vi "add search path.vi"(8 "error in":errorcluster, 10 "search path":path, 11 "glyph manager in":T1) -> (0 "error out":errorcluster, 3 "glyph manager out":T1)   [LabVIEW 2013, in "glyph manager.lvlib"]
uses:
  glyph manager.lvlib
  glyph manager.ctl
  <vilib>/picture/picture.llb/imagedata.ctl
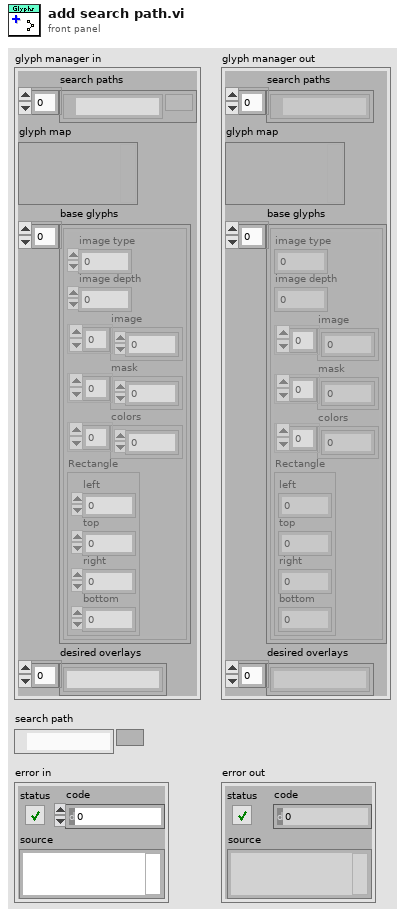
[diagram p1: front panel]
types:
  T1 = typedef "glyph manager.lvlib/glyph manager.ctl" = cluster{"search paths":path[], "glyph map":variant, "base glyphs":T2[], "desired overlays":string[]}
  T2 = typedef "imagedata.ctl" = cluster{"image type":i32, "image depth":i32, "image":u8[], "mask":u8[], "colors":u32[], "Rectangle":cluster{"left":i16, "top":i16, "right":i16, "bottom":i16}}
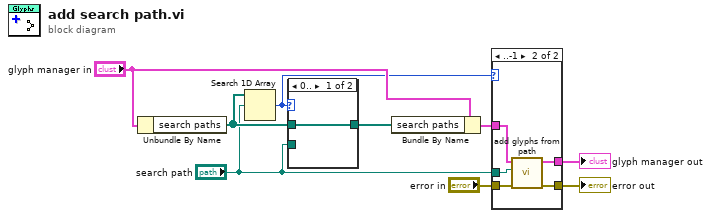
[diagram p0: block diagram]
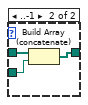
[diagram p3: hidden frame]
diagram:
  n1 = Unbundle By Name("glyph manager in") -> ("search paths"=w8:path[])
  n2 = Search 1D Array(1D array=w8, element="search path") -> (index of element=w5:i32)  [unwired: 1 in]
  n3 = case shown="0.." w5 {
    tunnel: w8 -> [w10 w13]
    tunnel: "search path" -> [_ w11]
    tunnel: [w10 w12] -> w7
    frame 0.. {
    }
    frame ..-1 {
      n4 = Build Array (concatenate)(w13, w11) -> (w12:path[])
    }
  }
  n5 = Bundle By Name(cluster="glyph manager in", "search paths"=w7) -> (w2:T1)
  n6 = case shown="..-1" w5 {
    tunnel: [w15 w20] -> w6
    tunnel: "error in" -> [w15 w19]
    tunnel: "search path" -> [_ w18]
    tunnel: w2 -> [w14 w17]
    tunnel: [w14 w16] -> w1
    frame 0.. {
    }
    frame ..-1 {
      n7 = call "add glyphs from path.vi"("error in (no error)"=w19, "Path"=w18, "glyph manager in"=w17) -> ("error out"=w20:errorcluster, "glyph manager out"=w16:T1)  [unwired: 7 in]
    }
  }
  "error out" <- w6
  "glyph manager out" <- w1
